vi "ChannelPropertiesHierarchy(non_numeric).vi"(11 "ChannelName":string) -> (3 "ElementsHierarchy":string[][](array[string]))   [LabVIEW 2013, in "TektronixDPO.lvclass"]
doc: "Return the properties hierarcy for the specified channel (only for NON numeric type properties)"
uses:
  TektronixDPO.lvclass
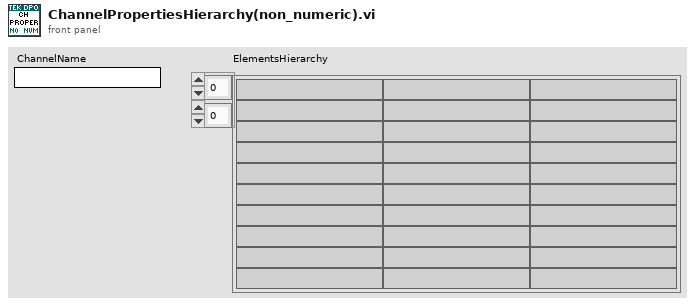
[diagram p1: front panel]
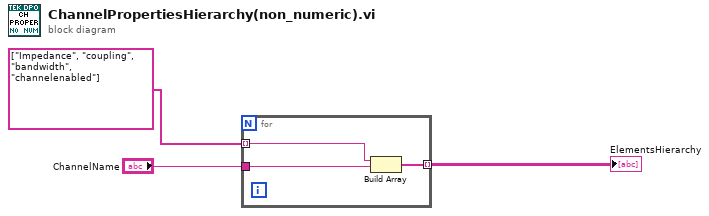
[diagram p0: block diagram]
diagram:
  n1 = for {
    tunnel: [w6] -> w3 mode=indexing
    tunnel: "ChannelName" -> [w5]
    tunnel: string[] ["Impedance", "coupling", "bandwidth", "channelenabled"] -> [w4] mode=indexing
    n2 = Build Array(w4, w5) -> (w6:string[])
  }
  "ElementsHierarchy" <- w3
